vi "get channels.vi"(11 "E2E configuration in":refnum<class "E2E Tag Exchange configuration.lvclass">) -> (2 "channels":refnum<class "TBM channel.lvclass">[](array[class]), 3 "E2E configuration out":refnum<class "E2E Tag Exchange configuration.lvclass">)   [LabVIEW 2015, in "E2E Tag Exchange configuration.lvclass"]
doc: "Returns an array of all Channels currently added to this configuration object."
uses:
  E2E Tag Exchange configuration.lvclass
  <vilib>/NI/Tag Bus Module Framework/channel/TBM channel.lvclass
  E2E Tag Exchange configuration.lvclass/E2E Tag Exchange configuration.ctl
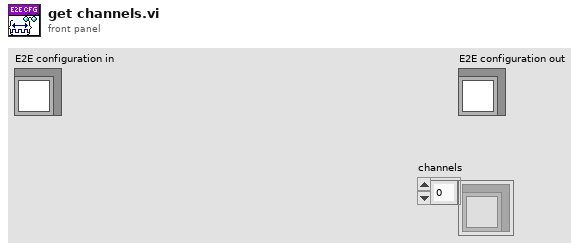
[diagram p1: front panel]
types:
  T1 = typedef "E2E Tag Exchange configuration.lvclass/Runtime Implementation.ctl" = enum16{"RT FIFO", "UDP"}
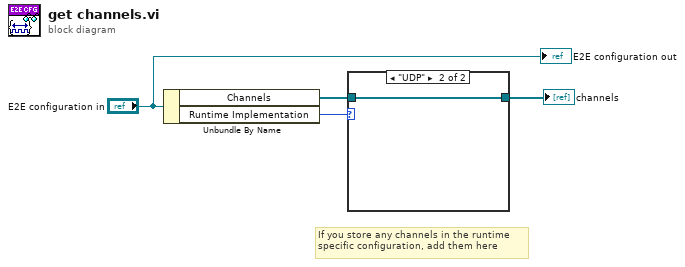
[diagram p0: block diagram]
diagram:
  # "If you store any channels in the runtime\nspecific configuration, add them here"
  n1 = Unbundle By Name("E2E configuration in") -> ("Channels"=w4:refnum<class "TBM channel.lvclass">[], "Runtime Implementation"=w3:T1)
  n2 = case shown="\"UDP\"" w3 {
    tunnel: w4 -> [w5 w6]
    tunnel: [w5 w6] -> w2
    frame "RT FIFO" {
    }
    frame "UDP" {
    }
  }
  "channels" <- w2
  "E2E configuration out" <- "E2E configuration in"
